vi "Sample_Coreset.vi"(8 "error in (no error)":errorcluster, 9 "coreset start idx":i32=-1, 10 "Sampling Ratio":sgl, 11 "Features (embeddings)":sgl[][](array[numeric])) -> (0 "error out":errorcluster, 1 "max distances":sgl[](array[numeric]), 2 "selected coreset idxs":i32[](array[numeric]), 3 "coreset":sgl[][](array[numeric]), 5 "dT_Coreset":dbl=0.00022729999909643084 format="%#_7f")   [LabVIEW 2020]
uses:
  <vilib>/Analysis/1siggen.llb/Ramp Pattern.vi
  <vilib>/Analysis/1siggen.llb/Ramp Pattern by Samples.vi
  Pairwise_Distance.vi
  Common/Array_2D_Reduce_Sum_Dim=1.vi
  <vilib>/addons/Multicore Analysis and Sparse Matrix/BLAS/gemv - General Matrix-Vector Product.vi
  <vilib>/addons/Multicore Analysis and Sparse Matrix/BLAS/_blas/sgemv - General Matrix-Vector Product (SGL).vi
  Progress Bar/API/ProgBar_Send.vi
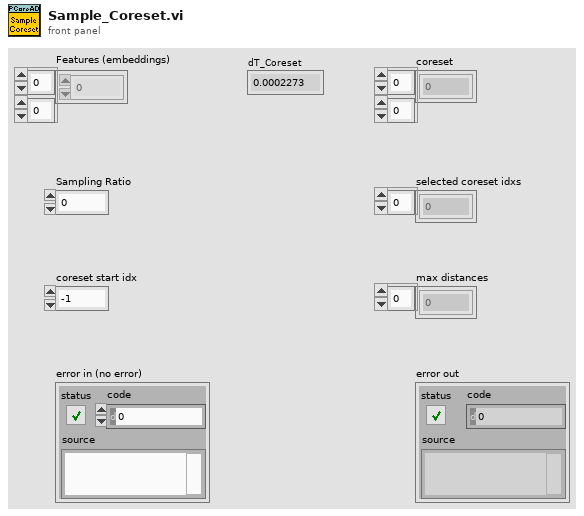
[diagram p1: front panel]
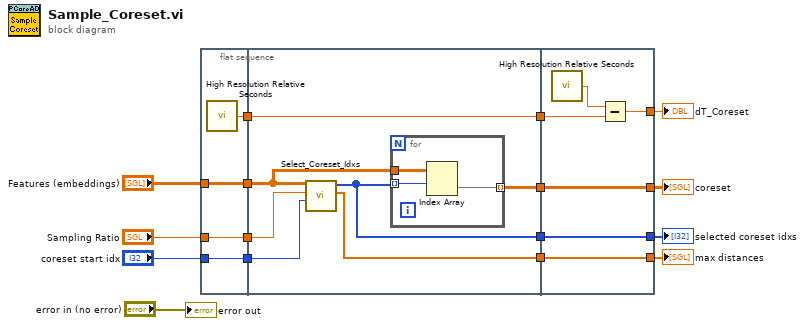
[diagram p0: block diagram]
diagram:
  n1 = flat-sequence {
    tunnel: "coreset start idx" -> [w18]
    tunnel: "Features (embeddings)" -> [w19]
    tunnel: "Sampling Ratio" -> [w20]
    tunnel: [w20] -> w12
    tunnel: [w19] -> w11
    tunnel: [w18] -> w10
    tunnel: [w17] -> w9
    tunnel: w12 -> [w27]
    tunnel: w11 -> [w26]
    tunnel: w10 -> [w25]
    tunnel: [w22] -> w8
    tunnel: [w24] -> w7
    tunnel: w9 -> [w24]
    tunnel: [w23] -> w4
    tunnel: [w21] -> w2
    tunnel: [w36] -> w14
    tunnel: w8 -> [w36]
    tunnel: w7 -> [w34]
    tunnel: [w33] -> w5
    tunnel: [w32] -> w3
    tunnel: w4 -> [w32]
    tunnel: [w31] -> w1
    tunnel: w2 -> [w31]
    frame #0 {
      n2 = call <vilib>:"High Resolution Relative Seconds.vi"() -> ("relative seconds"=w17:dbl)
    }
    frame #1 {
      n3 = call "Select_Coreset_Idxs.vi"("start idx"=w25, "Sampling Ratio"=w27, "Features (embeddings)"=w26) -> ("max distances"=w21:sgl[], "selected coreset idxs"=w23:i32[])  [unwired: 7 in]
      n4 = for {
        tunnel: w26 -> [w30]
        tunnel: w23 -> [w29] mode=indexing
        tunnel: [w28] -> w22 mode=indexing
        n5 = Index Array(array=w30, index (row)=w29) -> (element=w28:sgl[])  [unwired: 1 in]
      }
    }
    frame #2 {
      n6 = call <vilib>:"High Resolution Relative Seconds.vi"() -> ("relative seconds"=w35:dbl)
      n7 = Subtract(x=w35, y=w34) -> (x-y=w33:dbl)
    }
  }
  "coreset" <- w14
  "error out" <- "error in (no error)"
  "dT_Coreset" <- w5
  "selected coreset idxs" <- w3
  "max distances" <- w1
